vi "BotSpeak_GetVarVal.vi"(0 "Variable In":string="power", 1 "Bot Settings":T1) -> (2 "number":dbl, 4 "Bot Settings out":T1)   [LabVIEW 2012]
doc: "Retrieves the value of \"Variable in\" and returns that as \"value\". If the value is a number, this VI also returns that value in double format as \"number\"."
uses:
  <userlib>/BotSpeak/VIs/Direct/BotSpeak_Control.ctl
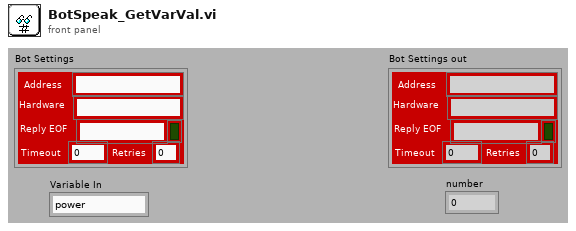
[diagram p1: front panel]
types:
  T1 = typedef "BotSpeak_Control.ctl" = cluster{"Address":string, "Reply EOF":string, "Hardware":string, "Retries":i8, "Timeout":i32, "Open?":bool}
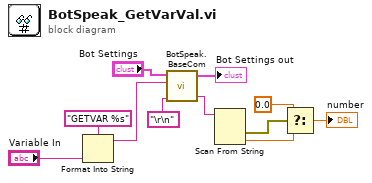
[diagram p0: block diagram]
diagram:
  n1 = Format Into String(format string="GETVAR %s" ("command"), "Variable In") -> (resulting string=w7:string)  [unwired: 2 in, 1 out]
  n2 = call <userlib>:"BotSpeak.BaseCom.vi"("Termination"="\r\n", "command"=w7, "Bot Settings in"="Bot Settings") -> ("response"=w1:string, "Bot Settings out"=→"Bot Settings out":T1)  [unwired: 2 in]
  n3 = Scan From String(input string=w1) -> (error out=w11:errorcluster, output 1=w9:dbl)  [unwired: 4 in, 2 out]
  n4 = Select(t=0.0, s=w11, f=w9) -> (s? t:f=→"number":dbl)
